vi "Lakeshore 331 write parameters to file.vi"(8 "error in (no error)":errorcluster, 11 "Lakeshore 331 in":refnum<class "Lakeshore 331.lvclass">) -> (0 "error out":errorcluster, 3 "Lakeshore 331 out":refnum<class "Lakeshore 331.lvclass">)   [LabVIEW 2022 SP3, in "Lakeshore 331.lvclass"]
uses:
  Lakeshore 331.lvclass
  Lakeshore 331.lvclass/Lakeshore 331.ctl
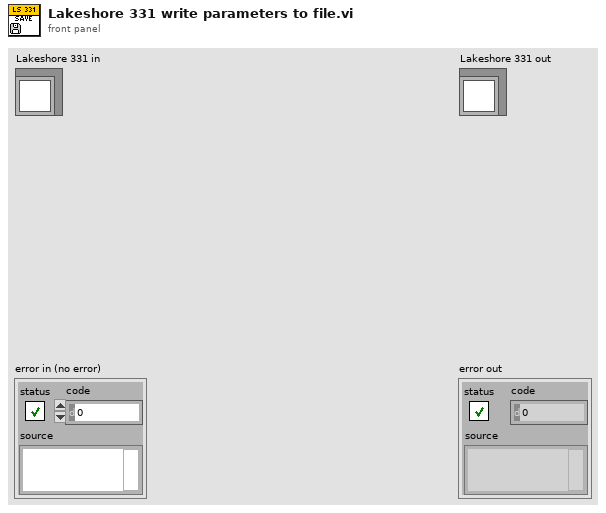
[diagram p1: front panel]
types:
  T1 = typedef "Lakeshore 331.lvclass/Lakeshore 331 Parameters.ctl" = cluster{"Mode":u16, "Setpoint":dbl, "Manual Power (%)":dbl, "Control Parameters":cluster{"P":dbl, "I":dbl, "D":u16}}
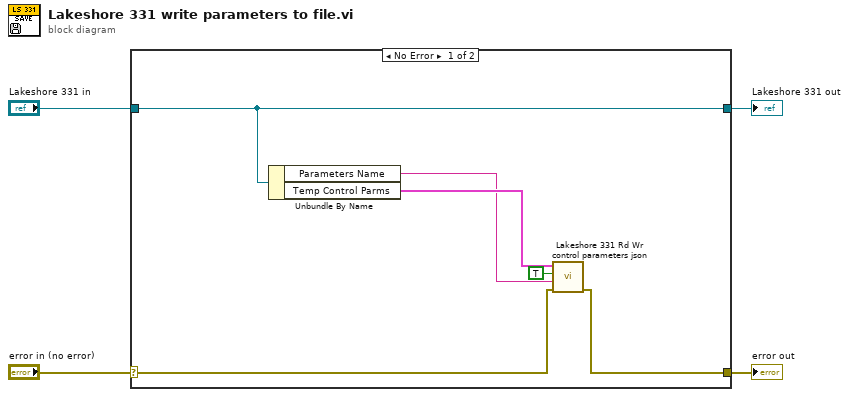
[diagram p0: block diagram]
diagram:
  n1 = case shown="No Error" "error in (no error)" {
    selector: "error in (no error)" -> [w6 w12]
    tunnel: [w5 w12] -> w3
    tunnel: [w7 w11] -> w1
    tunnel: "Lakeshore 331 in" -> [w7 w11]
    frame No Error {
      n2 = Unbundle By Name(w7) -> ("Parameters Name"=w9:string, "Temp Control Parms"=w10:T1)
      n3 = call "Lakeshore 331 Rd Wr control parameters json.vi"("error in (no error)"=w6, "Section"=w9, "Write? (F:Read)"=TRUE, "Temp Control Parms"=w10) -> ("error out"=w5:errorcluster)  [unwired: 6 in, 1 out]
    }
    frame Error {
    }
  }
  "error out" <- w3
  "Lakeshore 331 out" <- w1
